vi "DevWaitSync.vi"(8 "error in (no error)":errorcluster caption="entrée d'erreur (pas d'erreur)", 9 "Time in":u32, 10 "Type":enum16{"After", "Before"}(ring)=enum."Before", 11 "BaseDevice en entrée":refnum<class "BaseDevice.lvclass"> caption="DNL_LabVIEW Object in") -> (0 "error out":errorcluster caption="sortie d'erreur", 2 "Time":u32, 3 "BaseDevice en sortie":refnum<class "BaseDevice.lvclass"> caption="DNL_LabVIEW Object out")   [LabVIEW 2019, in "BaseDevice.lvclass"]
uses:
  BaseDevice.lvclass
  BaseDevice.lvclass/BaseDevice.ctl
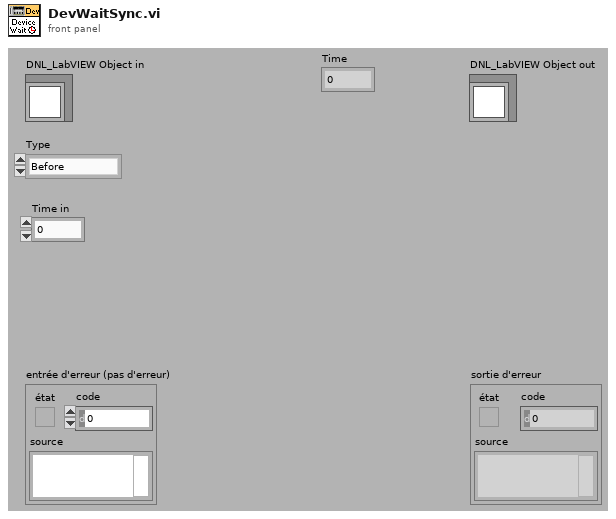
[diagram p1: front panel]
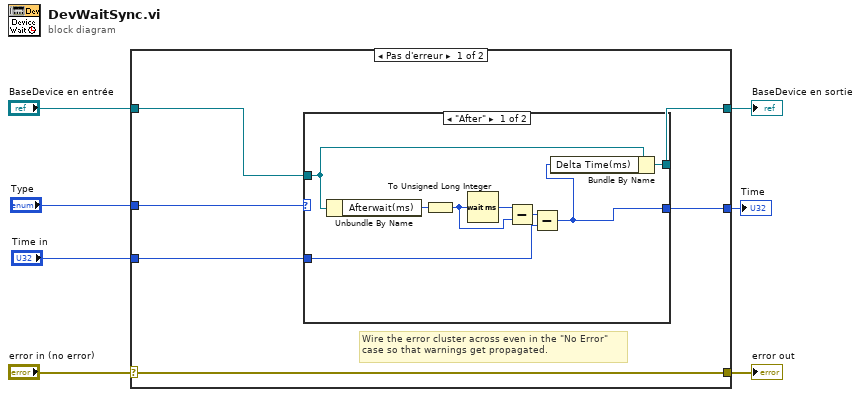
[diagram p0: block diagram]
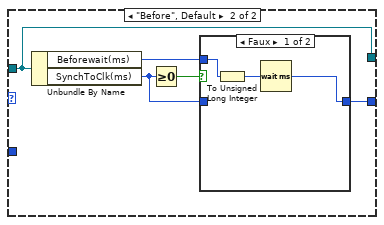
[diagram p2: hidden frame]
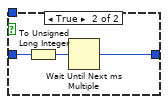
[diagram p3: hidden frame]
diagram:
  n1 = case shown="Pas d'erreur" "error in (no error)" {
    selector: "error in (no error)" -> [w13 w34]
    tunnel: [w13 w34] -> w6
    tunnel: [w8 w33] -> w4
    tunnel: "BaseDevice en entrée" -> [w11 w33]
    tunnel: "Type" -> [w12 _]
    tunnel: [w10 _] -> w2
    tunnel: "Time in" -> [w9 _]
    frame No Error {
      # "Wire the error cluster across even in the \"No Error\"\ncase so that warnings get propagated."
      n2 = case shown="\"After\"" w12 {
        tunnel: w11 -> [w16 w22]
        tunnel: [w14 w23] -> w10
        tunnel: w9 -> [w17 _]
        tunnel: [w15 w22] -> w8
        frame "After" {
          n3 = Unbundle By Name(w16) -> ("Afterwait(ms)"=w21:u32)
          n4 = To Unsigned Long Integer(number=w21) -> (unsigned 32bit integer=w19:u32)
          n5 = Wait (ms)(milliseconds to wait=w19) -> (millisecond timer value=w20:u32)
          n6 = Subtract(x=w20, y=w19) -> (x-y=w18:u32)
          n7 = Subtract(x=w18, y=w17) -> (x-y=w14:u32)
          n8 = Bundle By Name(cluster=w16, "Delta Time(ms)"=w14) -> (w15:refnum<class "BaseDevice.lvclass">)
        }
        frame "Before", Default {
          n9 = Unbundle By Name(w22) -> ("Beforewait(ms)"=w24:u32, "SynchToClk(ms)"=w25:i32)
          n10 = Greater Or Equal To 0?(x=w25) -> (x >= 0?=w26:bool)
          n11 = case shown="Faux" w26 {
            tunnel: w25 -> [_ w32]
            tunnel: w24 -> [w29 _]
            tunnel: [w27 w30] -> w23
            frame False {
              n12 = To Unsigned Long Integer(number=w29) -> (unsigned 32bit integer=w28:u32)
              n13 = Wait (ms)(milliseconds to wait=w28) -> (millisecond timer value=w27:u32)
            }
            frame True {
              n14 = To Unsigned Long Integer(number=w32) -> (unsigned 32bit integer=w31:u32)
              n15 = Wait Until Next ms Multiple(millisecond multiple=w31) -> (millisecond timer value=w30:u32)
            }
          }
        }
      }
    }
    frame Error {
    }
  }
  "error out" <- w6
  "BaseDevice en sortie" <- w4
  "Time" <- w2
